vi "Get Port Status.vi"(8 "Byte 0":string(combo), 9 "Byte 1":string(combo), 10 "CH":i32, 11 "Serial Devide Brand":T1) -> (2 "Expected Response":string, 3 "Command to Send":string)   [LabVIEW 2020]
uses:
  Combo Box Devices.ctl
  Combo Box Comandos.ctl
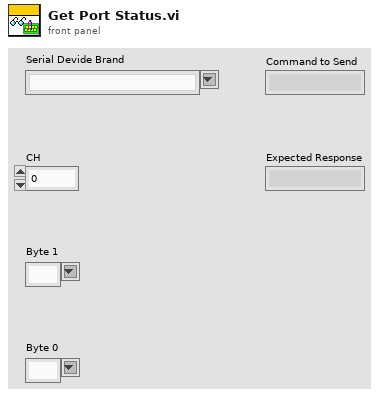
[diagram p1: front panel]
types:
  T1 = typedef "Combo Box Devices.ctl" = string
  T2 = typedef "Combo Box Comandos.ctl" = string
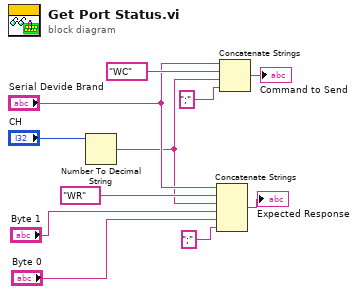
[diagram p0: block diagram]
diagram:
  n1 = Number To Decimal String(number="CH") -> (decimal integer string=w6:string)  [unwired: 1 in]
  n2 = Concatenate Strings("Serial Devide Brand", T2 "WR" ("Respuesta"), w6, "Byte 1", "Byte 0", ";" ("string")) -> (→"Expected Response":string)
  n3 = Concatenate Strings("Serial Devide Brand", T2 "WC" ("Command"), w6, ";" ("string")) -> (→"Command to Send":string)
